vi "Get Equation Variables.vi"(8 "error in (no error)":errorcluster, 11 "Format String":string) -> (0 "error out":errorcluster, 2 "Duplicate?":bool, 3 "Variables out":string[](array[string]))   [LabVIEW 2019, in "Instrument Addon Scripting API.lvlib"]
uses:
  Instrument Addon Scripting API.lvlib
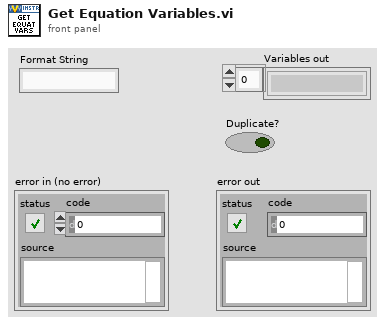
[diagram p1: front panel]
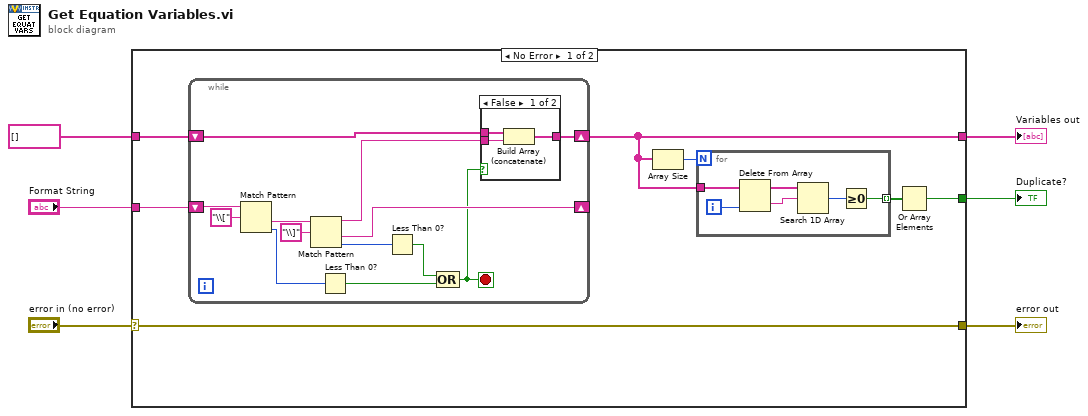
[diagram p0: block diagram]
diagram:
  n1 = case shown="No Error" "error in (no error)" {
    selector: "error in (no error)" -> [w11 w37]
    tunnel: "Format String" -> [w13 _]
    tunnel: string[] [] ("Array in") -> [w12 _]
    tunnel: [w8 _] -> w3
    tunnel: [w11 w37] -> w5
    tunnel: [w7 _] -> w6
    frame No Error {
      n2 = while {
        shift-right: [w28] -> _
        shift-left: w13 -> [w32]
        shift-right: [w21] -> w8
        shift-left: w12 -> [w23]
        stop <- w20 stop-if-true
        n3 = Match Pattern(string=w32, regular expression="\\[") -> (after substring=w30:string, offset past match=w26:i32)  [unwired: 1 in, 2 out]
        n4 = Match Pattern(string=w30, regular expression="\\]") -> (before substring=w22:string, after substring=w28:string, offset past match=w27:i32)  [unwired: 1 in, 1 out]
        n5 = Less Than 0?(x=w26) -> (x < 0?=w24:bool)
        n6 = Less Than 0?(x=w27) -> (x < 0?=w25:bool)
        n7 = Compound Arithmetic op=OR(w25, w24) -> (w20:bool)
        n8 = case shown="False" w20 {
          tunnel: w23 -> [w35 w36]
          tunnel: w22 -> [w34 _]
          tunnel: [w33 w36] -> w21
          frame False {
            n9 = Build Array (concatenate)(w35, w34) -> (w33:string[])
          }
          frame True {
          }
        }
      }
      n10 = Array Size(array=w8) -> (size(s)=w10:i32)
      n11 = for {
        N: w10 -> [_]
        tunnel: w8 -> [w19]
        tunnel: [w14] -> w9 mode=indexing
        i -> [w18]
        n12 = Delete From Array(array=w19, index=w18) -> (deleted portion=w16:string, array with subset deleted=w17:string[])  [unwired: 1 in]
        n13 = Search 1D Array(1D array=w17, element=w16) -> (index of element=w15:i32)  [unwired: 1 in]
        n14 = Greater Or Equal To 0?(x=w15) -> (x >= 0?=w14:bool)
      }
      n15 = Or Array Elements(Boolean array=w9) -> (logical OR=w7:bool)
    }
    frame Error {
    }
  }
  "Duplicate?" <- w6
  "error out" <- w5
  "Variables out" <- w3
